vi "GUI_USB Camera.vi"() -> ()   [LabVIEW 2013]
uses:
  Shared/GUI_Template/GUI_master/tcp_new_data_event.ctl
  Shared/GUI_Template/GUI_master/tcp new data cluster.ctl
panel:
  out "image::2":T1(plugin-control) caption="Image::2"
  in  "GUIdevice 2":string="PA2_Input2"
  in  "stop":bool
  out "image::1":T1(plugin-control) caption="USB Cam"
  in  "GUIdevice 1":string="PA2_Input1"
  out "tcp data event":T2
  out "error IO 2":errorcluster
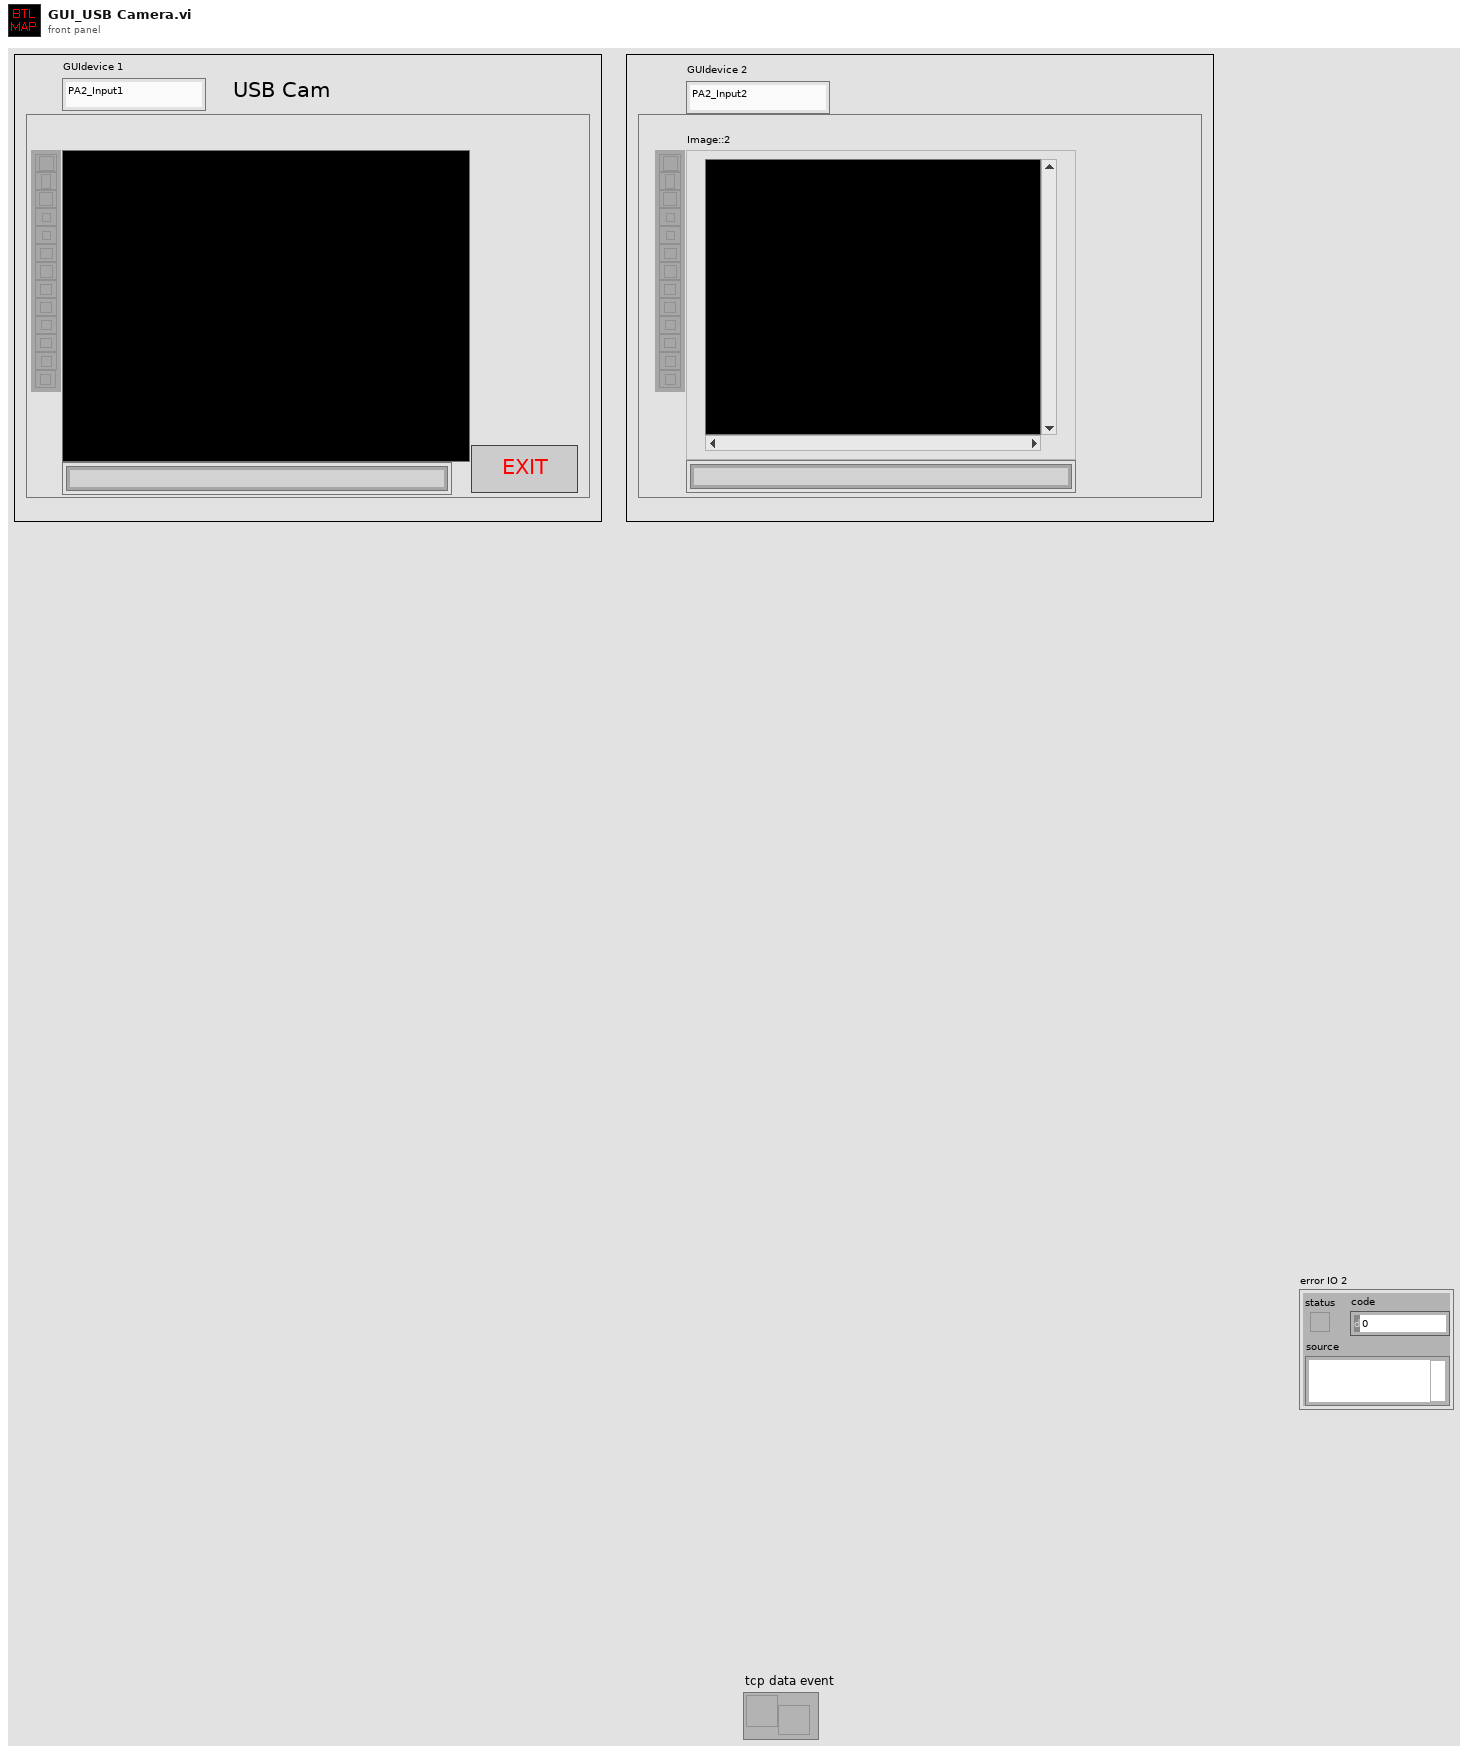
[diagram p1: front panel]
types:
  T1 = typedef "IMAQ Image.ctl" = refnum<image>
  T2 = typedef "tcp_new_data_event.ctl" = refnum<user-event>
  T3 = typedef "tcp new data cluster.ctl" = cluster{"EventEnum":enum16{"new data", "connection status update"}, "Device name":string}
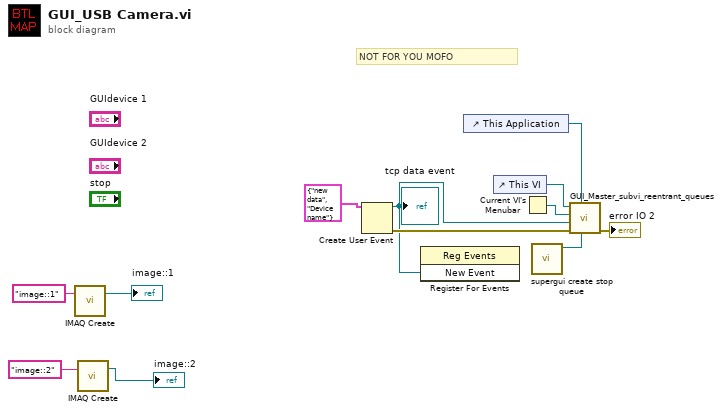
[diagram p0: block diagram]
diagram:
  # "NOT FOR YOU MOFO"
  n1 = call "IMAQ Create"("Image Name"="image::1") -> ("New Image"=→"image::1":T1)  [unwired: 4 in, 1 out]
  n2 = call "IMAQ Create"("Image Name"="image::2") -> ("New Image"=→"image::2":T1)  [unwired: 4 in, 1 out]
  n3 = Create User Event(user event datatype=T3 {"EventEnum"=enum."new data", "Device name"="Device name"} ("New Event")) -> (user event=w7:refnum<user-event>, error out=w8:errorcluster)  [unwired: 1 in]
  "tcp data event" <- w7
  n4 = register-events(w7) -> ()  [unwired: 2 in, 2 out]
  n5 = control-ref of="This Application"() -> (w6:refnum<vi>)
  n6 = control-ref of="This VI"() -> (w11:refnum<vi>)
  n7 = Current VI's Menubar() -> (w10:refnum<k9>)
  n8 = call "supergui create stop queue.vi"() -> ("STOP Queue out"=w1:refnum<queue>)  [unwired: 11 in]
  n9 = call "GUI_Master_subvi_reentrant_queues.vi"("STOP Queue in"=w1, "This Application"=w6, "error in (no error)"=w8, "tcp data event"=w7, "Caller menu reference"=w10, "Caller VI ref"=w11) -> ("error out"=→"error IO 2":errorcluster)  [unwired: 5 in]
